vi "Read Vertical Scrollbar Visible.vi"(9 "Array in":refnum<class "Array.lvclass">) -> (3 "Array out":refnum<class "Array.lvclass">, 4 "Vertical Scrollbar Visible":bool)   [LabVIEW 2014, in "Array.lvclass"]
uses:
  Array.lvclass
  Array.lvclass/Array.ctl
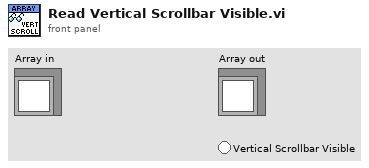
[diagram p1: front panel]
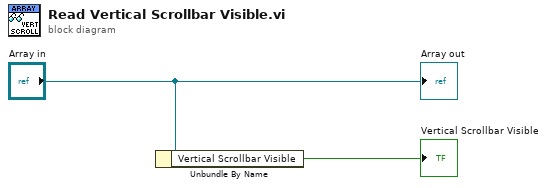
[diagram p0: block diagram]
diagram:
  n1 = Unbundle By Name("Array in") -> ("Vertical Scrollbar Visible"=→"Vertical Scrollbar Visible":bool)
  "Array out" <- "Array in"
